vi "Grab and Select Interface.vi"() -> ()   [LabVIEW 2011]
doc: "The Grab and Select Interface VI acquires images continuously and displays the images in an image control using high-level acquisition VIs. This example also demonstrates the capability to enumerate the available interfaces and dynamically change which camera to acquire from. A grab is appropriate for high-speed applications in which you need to process only one image at a time."
uses:
  <vilib>/vision/driver/NI_Vision_Acquisition_Software.lvlib
panel:
  out "Frame Rate":dbl(knob) scale=0.0..100.0
  out "Buffer Number":u32
  out "Image":T1(plugin-control)
  in  "Stop":bool
  in  "Interfaces":i32(listbox)
  # "Overview: Demonstrates how to enumerate the available cameras, and dynamically change which camera to acquire from.\nRequirements: Vision Acquisition Software, multiple cameras\nInstructions: \n1. Run the VI\n2. Select one of the available Interfaces."
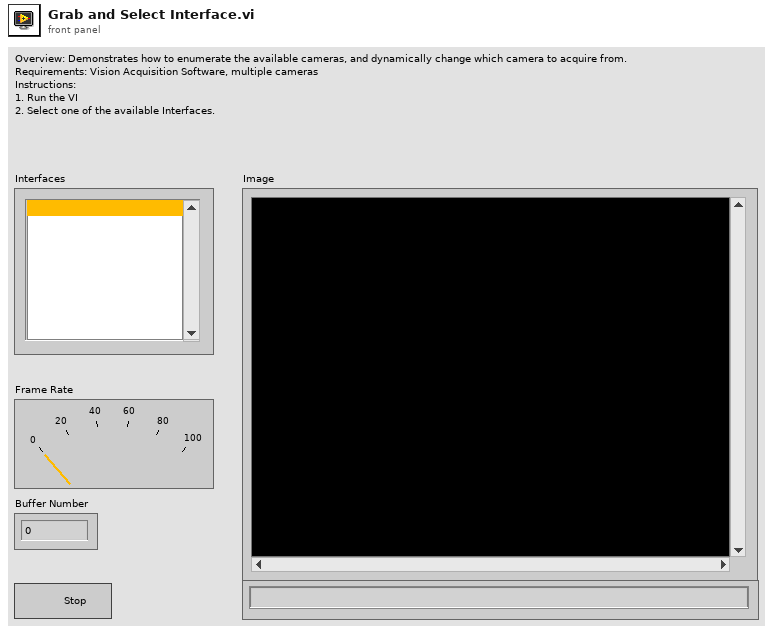
[diagram p1: front panel]
types:
  T1 = typedef "IMAQ Image.ctl" = refnum<image>
  T2 = cluster{"Type":u32, "Version":u32, "Flags":u32, "SerialNumberHigh":u32, "SerialNumberLow":u32, "BusType":u32, "InterfaceName":string, "VendorName":string, "ModelName":string, "CameraFileName":string, "CameraAttributeURL":string}[]
  T3 = typedef "IMAQdx.ctl" = refnum<k21>
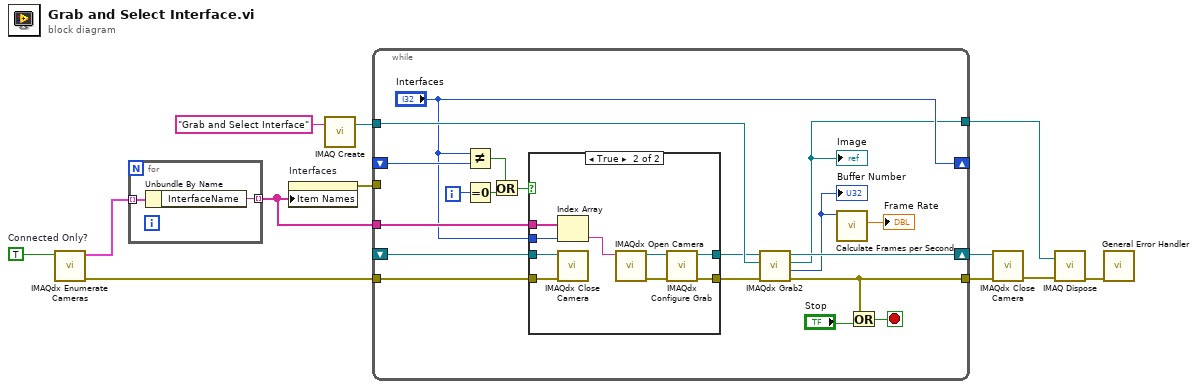
[diagram p0: block diagram]
diagram:
  w5 = TRUE  # Connected Only?
  n1 = call <vilib>:"IMAQdx Enumerate Cameras.vi"("Connected Only? (Yes)"=w5) -> ("error out"=w11:errorcluster, "Camera Information Array"=w6:T2)  [unwired: 1 in, 8 out]
  n2 = for {
    tunnel: w6 -> [w14] mode=indexing
    tunnel: [w13] -> w4 mode=indexing
    n3 = Unbundle By Name(w14) -> ("InterfaceName"=w13:string)
  }
  n4 = property on="Interfaces" class="LstBox (strict)"("Item Names"=w4) -> (error out=w7:errorcluster)  [unwired: 2 in, 1 out]
  n5 = call "IMAQ Create"("Image Name"="Grab and Select Interface") -> ("New Image"=w9:T1)  [unwired: 3 in, 2 out]
  n6 = while {
    shift-left: _ -> [w29]
    shift-right: ["Interfaces"] -> _
    tunnel: w9 -> [w32]
    tunnel: w11 -> [w33]
    tunnel: [w16] -> w12
    tunnel: w4 -> [w22]
    shift-right: [w23] -> w8
    shift-left: _ -> [w20]
    tunnel: w7 -> [_]
    tunnel: [w15] -> w3
    i -> [w26]
    stop <- w30 stop-if-true
    n7 = Not Equal?(x="Interfaces", y=w29) -> (x != y?=w27:bool)
    n8 = Equal To 0?(x=w26) -> (x = 0?=w25:bool)
    n9 = Or(x=w27, y=w25) -> (x .or. y?=w28:bool)
    n10 = case shown="True" w28 {
      tunnel: w33 -> [w35 w37]
      tunnel: [w35 w40] -> w24
      tunnel: "Interfaces" -> [_ w44]
      tunnel: w22 -> [_ w43]
      tunnel: [w34 w38] -> w21
      tunnel: w20 -> [w34 w42]
      frame False {
      }
      frame True {
        n11 = Index Array(array=w43, index=w44) -> (element=w36:string)
        n12 = call <vilib>:"IMAQdx Close Camera.vi"("error in"=w37, "Session In"=w42) -> ()  [unwired: 10 out]
        n13 = call <vilib>:"IMAQdx Open Camera.vi"("Session In"=w36) -> ("error out"=w41:errorcluster, "Session Out"=w39:T3)  [unwired: 2 in, 7 out]
        n14 = call <vilib>:"IMAQdx Configure Grab.vi"("error in"=w41, "Session In"=w39) -> ("error out"=w40:errorcluster, "Session Out"=w38:T3)  [unwired: 8 out]
      }
    }
    n15 = call <vilib>:"IMAQdx Grab2.vi"("error in"=w24, "Image In"=w32, "Session In"=w21) -> ("error out"=w16:errorcluster, "Buffer Number Out"=w18:u32, "Image Out"=w15:T1, "Session Out"=w23:T3)  [unwired: 5 in]
    "Image" <- w15
    "Buffer Number" <- w18
    n16 = call <vilib>:"Calculate Frames per Second.vi"("Buffer Number"=w18) -> ("Processed Frames/s"=→"Frame Rate":dbl)  [unwired: 8 in, 2 out]
    n17 = Or(x=w16, y="Stop") -> (x .or. y?=w30:bool)
  }
  n18 = call <vilib>:"IMAQdx Close Camera.vi"("error in"=w12, "Session In"=w8) -> ("error out"=w2:errorcluster)  [unwired: 9 out]
  n19 = call "IMAQ Dispose"("Image"=w3, "error in (no error)"=w2) -> ("error out"=w1:errorcluster)  [unwired: 4 in]
  n20 = call <vilib>:"General Error Handler.vi"("error in (no error)"=w1) -> ()  [unwired: 1 in, 14 out]
